vi "GetErrorUXFromError.vi"(8 "error in (no error)":errorcluster) -> (0 "error out":errorcluster, 3 "ErrorUX":T1)   [LabVIEW 2019, in "LabErrorUX.lvclass"]
uses:
  LabErrorUX.lvclass
  Typedefs/ErrorUX.ctl
  <vilib>/SLL Toolkit/SLL String/SLL String.lvlib
  <vilib>/SLL Toolkit/SLL String/_SubVIs/I32 to String.vi
panel:
  out "Map":map{string, string}(c390)
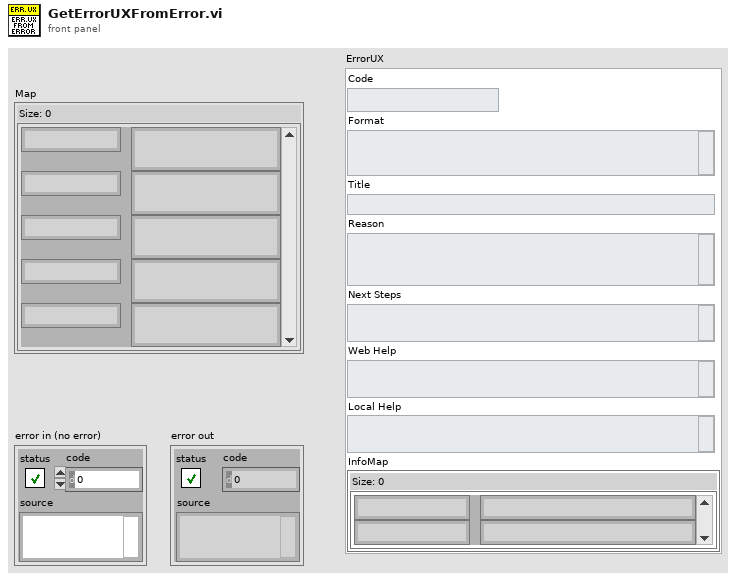
[diagram p1: front panel]
types:
  T1 = typedef "LabErrorUX.lvclass/ErrorUX.ctl" = cluster{"Code":string, "Format":string, "Title":string, "Reason":string, "Next Steps":string, "Web Help":string, "Local Help":string, "InfoMap":map{string, string}}
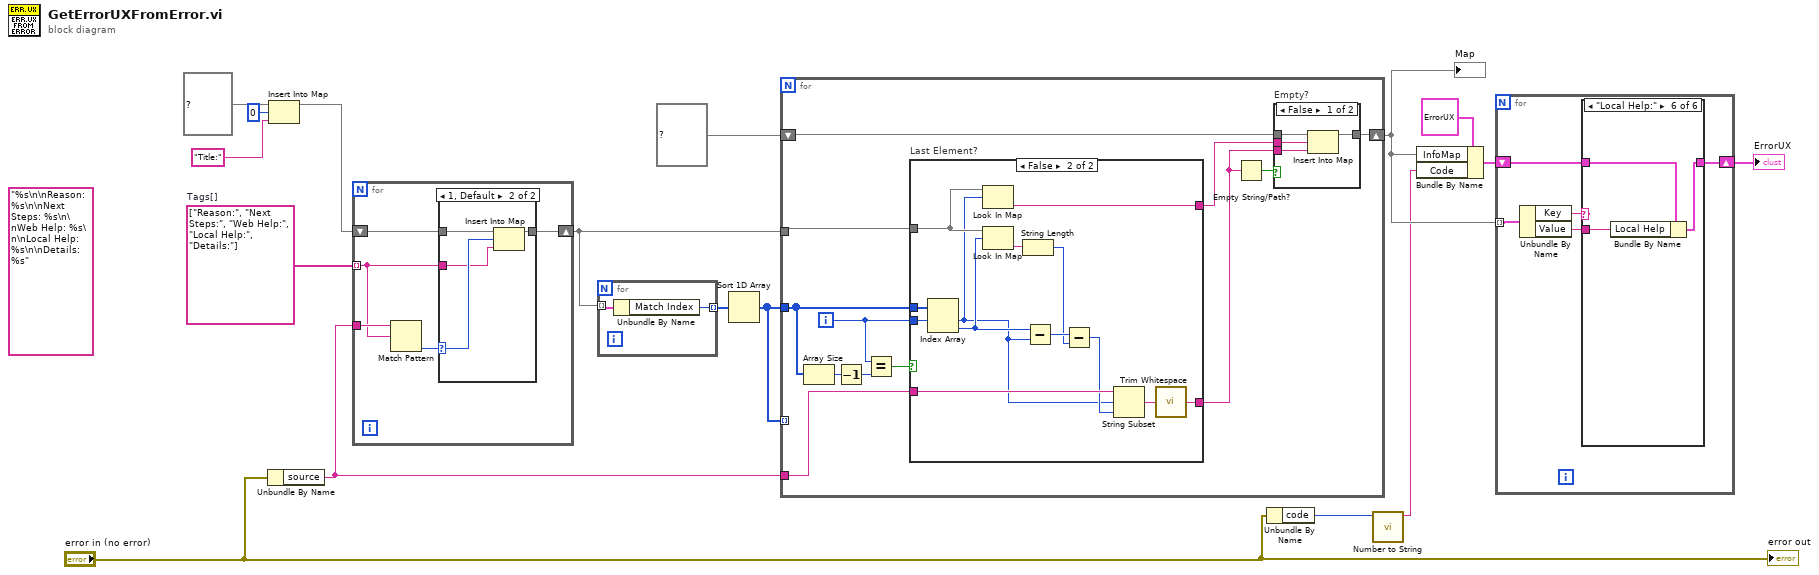
[diagram p0: block diagram]
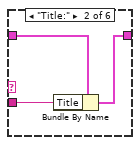
[diagram p3: hidden frame]
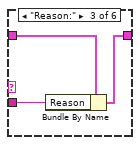
[diagram p4: hidden frame]
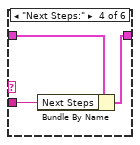
[diagram p5: hidden frame]
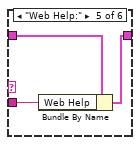
[diagram p6: hidden frame]
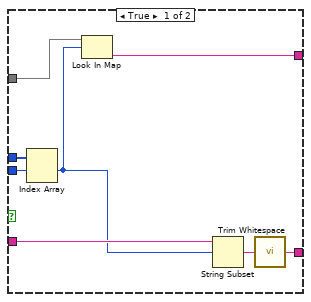
[diagram p8: hidden frame]
diagram:
  w17 = string[] ["Reason:", "Next Steps:", "Web Help:", "Local Help:", "Details:"]  # Tags[]
  (unwired) "%s\n\nReason: %s\n\nNext Steps: %s\n\nWeb Help: %s\n\nLocal Help: %s\n\nDetails: %s" ("format string")
  n1 = Unbundle By Name("error in (no error)") -> ("source"=w15:string)
  n2 = Insert Into Map(map in=map{i32, string} {} ("map"), key=0, value="Title:") -> (map out=w13:map{i32, string})  [unwired: 2 out]
  n3 = for {
    tunnel: w17 -> [w18] mode=indexing
    tunnel: w15 -> [w22]
    shift-right: [w21] -> w6
    shift-left: w13 -> [w20]
    n4 = Match Pattern(string=w22, regular expression=w18) -> (offset past match=w19:i32)  [unwired: 1 in, 3 out]
    n5 = case shown="1, Default" w19 {
      selector: w19 -> [_ w26]
      tunnel: [w23 w27] -> w21
      tunnel: w18 -> [_ w25]
      tunnel: w20 -> [w23 w24]
      frame -1 {
      }
      frame 1, Default {
        n6 = Insert Into Map(map in=w24, key=w26, value=w25) -> (map out=w27:map{i32, string})  [unwired: 2 out]
      }
    }
  }
  n7 = for {
    tunnel: w6 -> [w29] mode=indexing
    tunnel: [w28] -> w4 mode=indexing
    n8 = Unbundle By Name(w29) -> ("Match Index"=w28:i32)
  }
  n9 = Sort 1D Array(array=w4) -> (sorted array=w16:i32[])
  n10 = for {
    tunnel: w16 -> [_] mode=indexing
    tunnel: w15 -> [w41]
    tunnel: w6 -> [w40]
    tunnel: w16 -> [w36]
    shift-right: [w38] -> w8
    shift-left: map{string, string} {} ("map") -> [w37]
    i -> [w33]
    n11 = Array Size(array=w36) -> (size(s)=w35:i32)
    n12 = Decrement(x=w35) -> (x-1=w34:i32)
    n13 = Equal?(x=w33, y=w34) -> (x = y?=w32:bool)
    n14 = case "Last Element?" shown="False" w32 {
      tunnel: w41 -> [w54 w67]
      tunnel: w40 -> [w53 w61]
      tunnel: [w51 w59] -> w39
      tunnel: [w49 w57] -> w31
      tunnel: w36 -> [w48 w56]
      tunnel: w33 -> [w47 w55]
      frame True {
        n15 = Index Array(array=w48, index #1=w47) -> (element #1=w52:i32)  [unwired: 1 in, 1 out]
        n16 = Look In Map(map=w53, key=w52) -> (value=w51:string)  [unwired: 1 in, 1 out]
        n17 = String Subset(string=w54, offset (0)=w52) -> (substring=w50:string)  [unwired: 1 in]
        n18 = call <vilib>:"Trim Whitespace.vi"("string"=w50) -> ("trimmed string"=w49:string)  [unwired: 1 in]
      }
      frame False {
        n19 = Index Array(array=w56, index #1=w55) -> (element #1=w60:i32, element #2=w65:i32)  [unwired: 1 in]
        n20 = Look In Map(map=w61, key=w60) -> (value=w59:string)  [unwired: 1 in, 1 out]
        n21 = Look In Map(map=w61, key=w65) -> (value=w66:string)  [unwired: 1 in, 1 out]
        n22 = String Length(string=w66) -> (length=w63:i32)
        n23 = Subtract(x=w65, y=w60) -> (x-y=w64:i32)
        n24 = Subtract(x=w64, y=w63) -> (x-y=w62:i32)
        n25 = String Subset(string=w67, offset (0)=w60, length (rest)=w62) -> (substring=w58:string)
        n26 = call <vilib>:"Trim Whitespace.vi"("string"=w58) -> ("trimmed string"=w57:string)  [unwired: 1 in]
      }
    }
    n27 = Empty String/Path?(string/path=w31) -> (empty?=w30:bool)
    n28 = case "Empty?" shown="False" w30 {
      tunnel: w39 -> [w45 _]
      tunnel: [w44 w46] -> w38
      tunnel: w37 -> [w43 w46]
      tunnel: w31 -> [w42 _]
      frame False {
        n29 = Insert Into Map(map in=w43, key=w45, value=w42) -> (map out=w44:map{string, string})  [unwired: 2 out]
      }
      frame True {
      }
    }
  }
  "Map" <- w8
  n30 = Unbundle By Name("error in (no error)") -> ("code"=w2:i32)
  n31 = call-poly <vilib>:"Number to String.vi"("Numeric"=w2) -> ("String"=w1:string)  [unwired: 10 in]
  n32 = Bundle By Name(cluster=T1 {"Code"="", "Format"="", "Title"="", "Reason"="", "Next Steps"="", "Web Help"="", "Local Help"="", "InfoMap"={}} ("ErrorUX"), "InfoMap"=w8, "Code"=w1) -> (w7:T1)
  n33 = for {
    tunnel: w8 -> [w72] mode=indexing
    shift-right: [w68] -> w10
    shift-left: w7 -> [w69]
    n34 = Unbundle By Name(w72) -> ("Key"=w71:string, "Value"=w70:string)
    n35 = case shown="\"Local Help:\"" w71 {
      tunnel: w70 -> [_ w74 w77 w80 w83 w86]
      tunnel: w69 -> [w73 w76 w79 w82 w85 w88]
      tunnel: [w73 w75 w78 w81 w84 w87] -> w68
      frame Default {
      }
      frame "Title:" {
        n36 = Bundle By Name(cluster=w76, "Title"=w74) -> (w75:T1)
      }
      frame "Reason:" {
        n37 = Bundle By Name(cluster=w79, "Reason"=w77) -> (w78:T1)
      }
      frame "Next Steps:" {
        n38 = Bundle By Name(cluster=w82, "Next Steps"=w80) -> (w81:T1)
      }
      frame "Web Help:" {
        n39 = Bundle By Name(cluster=w85, "Web Help"=w83) -> (w84:T1)
      }
      frame "Local Help:" {
        n40 = Bundle By Name(cluster=w88, "Local Help"=w86) -> (w87:T1)
      }
    }
  }
  "ErrorUX" <- w10
  "error out" <- "error in (no error)"
